vi "RT_DMARS (SubVI).vi"(5 "y2":dbl[](array[numeric]), 7 "y1":dbl[](array[numeric]), 9 "u3":dbl[](array[numeric]), 10 "u2":dbl[](array[numeric]), 11 "u1":dbl[](array[numeric])) -> (3 "DMARS Data":dbl[](array[numeric]))   [LabVIEW 2017]
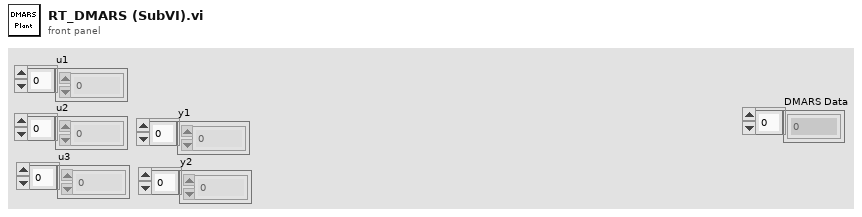
[diagram p1: front panel]
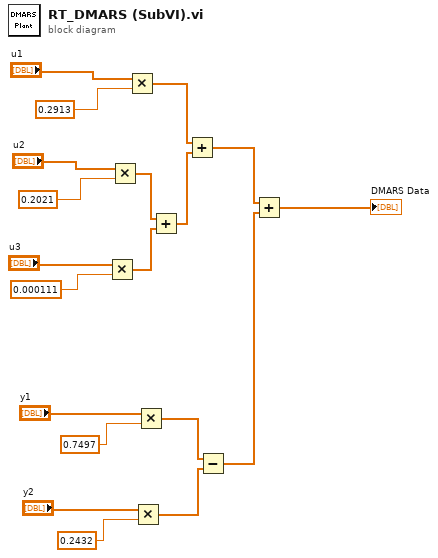
[diagram p0: block diagram]
diagram:
  n1 = Multiply(x="u3", y=0.000111) -> (x*y=w12:dbl[])
  n2 = Multiply(x="u2", y=0.2021) -> (x*y=w13:dbl[])
  n3 = Multiply(x="u1", y=0.2913) -> (x*y=w8:dbl[])
  n4 = Multiply(x="y2", y=0.2432) -> (x*y=w16:dbl[])
  n5 = Multiply(x="y1", y=0.7497) -> (x*y=w17:dbl[])
  n6 = Add(x=w13, y=w12) -> (x+y=w7:dbl[])
  n7 = Add(x=w8, y=w7) -> (x+y=w6:dbl[])
  n8 = Subtract(x=w17, y=w16) -> (x-y=w11:dbl[])
  n9 = Add(x=w6, y=w11) -> (x+y=→"DMARS Data":dbl[])
